vi "VCA_XS.vi"(6 "EG":fxp<+,8,0>=0.99609375, 9 "Sample In":fxp<+/-,18,18>) -> (1 "Sample Out":fxp<+/-,18,18>)   [LabVIEW 2015]
doc: "Attenuates an input sample when 'EG' < 1.\n\nThe latency of this VI is 7 cycles."
uses:
  <vilib>/rvi/FXPMathLib/FxpMul/XNode/nifxpmath_Multiplier.xnode
  <vilib>/rvi/FXPMathLib/sim/FxpSim.dll
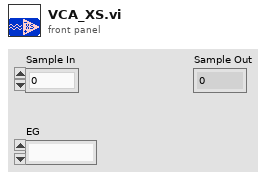
[diagram p1: front panel]
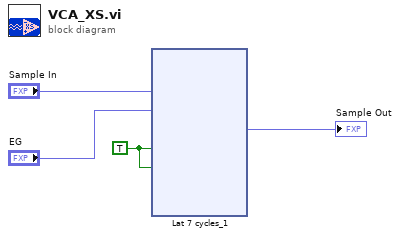
[diagram p0: block diagram]
diagram:
  w2 = TRUE ("input valid")
  n1 = xnode "Lat 7 cycles_1"("x"="Sample In", "y"="EG", "input valid"=w2, "ready for output (T)"=w2) -> ("x*y"=→"Sample Out":fxp<+/-,18,18>)  [unwired: 2 out]
